vi "play.vi"(8 "error in (no error)":errorcluster, 11 "Game in":refnum<class "Game.lvclass">) -> (0 "error out":errorcluster, 3 "Game out":refnum<class "Game.lvclass">)   [LabVIEW 2018, in "Game.lvclass"]
uses:
  Game.lvclass
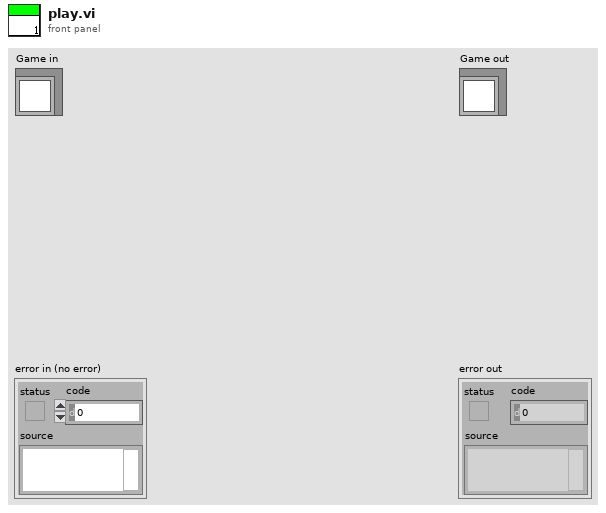
[diagram p1: front panel]
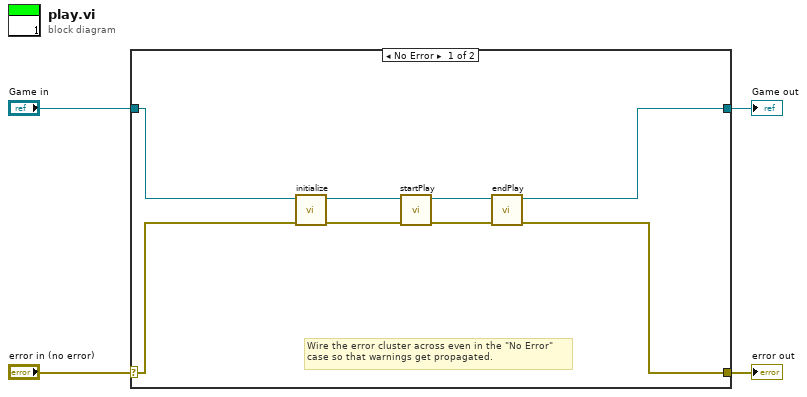
[diagram p0: block diagram]
diagram:
  n1 = case shown="No Error" "error in (no error)" {
    selector: "error in (no error)" -> [w12 w14]
    tunnel: [w7 w14] -> w3
    tunnel: [w5 w13] -> w1
    tunnel: "Game in" -> [w10 w13]
    frame No Error {
      # "Wire the error cluster across even in the \"No Error\"\ncase so that warnings get propagated."
      n2 = call-dynamic "initialize.vi"("error in (no error)"=w12, "Game in"=w10) -> ("error out"=w11:errorcluster, "Game out"=w8:refnum<class "Game.lvclass">)  [unwired: 8 in]
      n3 = call-dynamic "startPlay.vi"("error in (no error)"=w11, "Game in"=w8) -> ("error out"=w9:errorcluster, "Game out"=w6:refnum<class "Game.lvclass">)  [unwired: 8 in]
      n4 = call-dynamic "endPlay.vi"("error in (no error)"=w9, "Game in"=w6) -> ("error out"=w7:errorcluster, "Game out"=w5:refnum<class "Game.lvclass">)  [unwired: 8 in]
    }
    frame Error {
    }
  }
  "error out" <- w3
  "Game out" <- w1
